vi "SUB_RTXDll_ReadWait.vi"(3 "CMD":string) -> (1 "OUTPUT":string)   [LabVIEW 2011]
uses:
  R2012dll.dll
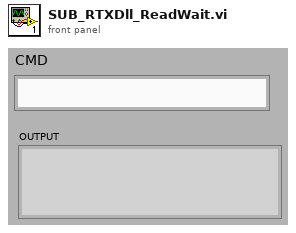
[diagram p1: front panel]
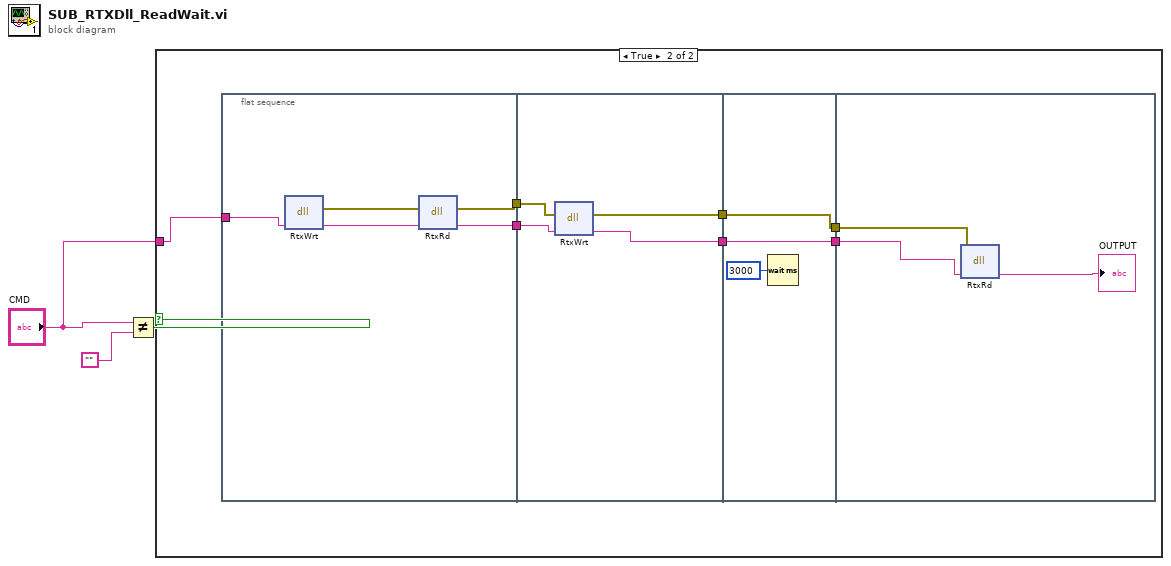
[diagram p0: block diagram]
diagram:
  n1 = Not Equal?(x="CMD", y="") -> (x != y?=w2:bool)
  n2 = case shown="True" w2 {
    tunnel: "CMD" -> [_ w10]
    frame False {
    }
    frame True {
      n3 = flat-sequence {
        tunnel: w10 -> [w15]
        tunnel: [w12] -> w9
        tunnel: [w11] -> w8
        tunnel: w9 -> [w19]
        tunnel: w8 -> [w18]
        tunnel: [w17] -> w6
        tunnel: [w16] -> w4
        tunnel: [w21] -> w7
        tunnel: w6 -> [w21]
        tunnel: [w20] -> w5
        tunnel: w4 -> [w20]
        tunnel: w7 -> [w24]
        tunnel: w5 -> [w23]
        frame #0 {
          n4 = dll-call lib="E:/Konftel_Project/R2012dll.dll" fn="RtxWrt"("RtxWrt"=w15) -> (error out=w14:errorcluster, "RtxWrt"=w13:string)  [unwired: 4 in, 1 out]
          n5 = dll-call lib="E:/Konftel_Project/R2012dll.dll" fn="RtxRd"(error in=w14, "RtxRd"=w13) -> (error out=w11:errorcluster, "RtxRd"=w12:string)  [unwired: 3 in, 1 out]
        }
        frame #1 {
          n6 = dll-call lib="E:/Konftel_Project/R2012dll.dll" fn="RtxWrt"(error in=w18, "RtxWrt"=w19) -> (error out=w17:errorcluster, "RtxWrt"=w16:string)  [unwired: 3 in, 1 out]
        }
        frame #2 {
          n7 = Wait (ms)(milliseconds to wait=u32 3000) -> ()  [unwired: 1 out]
        }
        frame #3 {
          n8 = dll-call lib="E:/Konftel_Project/R2012dll.dll" fn="RtxRd"(error in=w24, "RtxRd"=w23) -> ("RtxRd"=→"OUTPUT":string)  [unwired: 3 in, 2 out]
        }
      }
    }
  }
